vi "Flatten.vi"(8 "error in":errorcluster, 9 "Data":T1) -> (0 "error out":errorcluster, 2 "Buffer":u8[](array[numeric]) format="%.0x")   [LabVIEW 2020, in "TcpClientHello.lvlib"]
uses:
  TcpClientHello.lvlib
  Data.ctl
  lv-protoc/LV-Proto/Wire Encode Tag.vi
  lv-protoc/LV-Proto/Encode bytes.vi
  lv-protoc/LV-Proto/Wire Encode Varint I32.vi
  lv-protoc/LV-Proto/Encode LEN.vi
  lv-protoc/LV-Proto/LV-Proto.lvlib
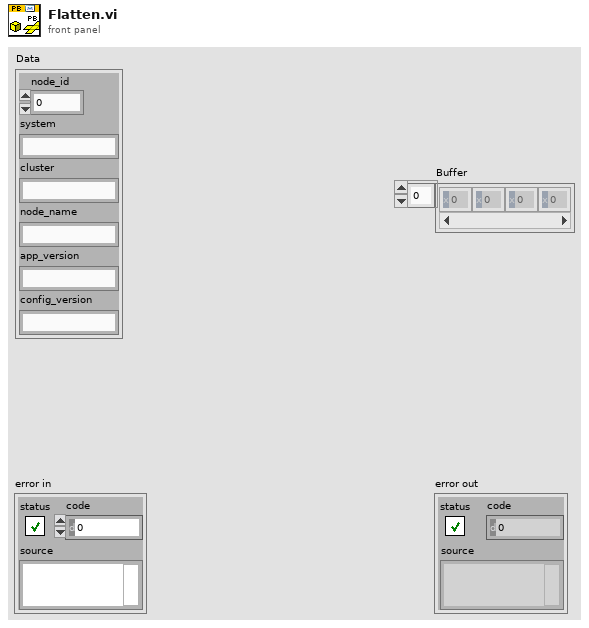
[diagram p1: front panel]
types:
  T1 = typedef "TcpClientHello.lvlib/Data.ctl" = cluster{"node_id":u32, "system":string, "cluster":string, "node_name":string, "app_version":string, "config_version":string}
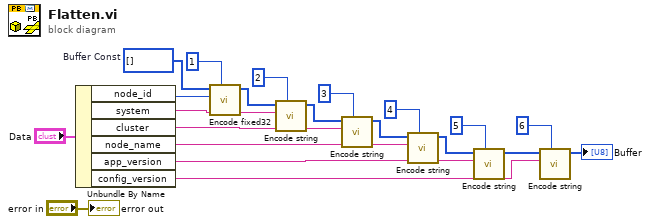
[diagram p0: block diagram]
diagram:
  w19 = u8[] []  # Buffer Const
  n1 = Unbundle By Name("Data") -> ("node_id"=w17:u32, "system"=w14:string, "cluster"=w11:string, "node_name"=w8:string, "app_version"=w5:string, "config_version"=w2:string)
  n2 = call "Encode fixed32.vi"("Field Number"=1, "fixed32"=w17, "Buffer in"=w19) -> ("Buffer"=w16:u8[])  [unwired: 8 in]
  n3 = call "Encode string.vi"("Field Number"=2, "string"=w14, "Buffer in"=w16) -> ("Buffer"=w13:u8[])  [unwired: 8 in]
  n4 = call "Encode string.vi"("Field Number"=3, "string"=w11, "Buffer in"=w13) -> ("Buffer"=w10:u8[])  [unwired: 8 in]
  n5 = call "Encode string.vi"("Field Number"=4, "string"=w8, "Buffer in"=w10) -> ("Buffer"=w7:u8[])  [unwired: 8 in]
  n6 = call "Encode string.vi"("Field Number"=5, "string"=w5, "Buffer in"=w7) -> ("Buffer"=w4:u8[])  [unwired: 8 in]
  n7 = call "Encode string.vi"("Field Number"=6, "string"=w2, "Buffer in"=w4) -> ("Buffer"=→"Buffer":u8[])  [unwired: 8 in]
  "error out" <- "error in"
